vi "Update Configuration Ctls.vi"(6 "Units":refnum<vi>, 8 "error in":errorcluster, 9 "Type":refnum<vi>, 10 "selected channels":i32[](listbox)=[0], 11 "9210 in":refnum<class "9210.lvclass">) -> (0 "error out":errorcluster, 3 "9210 out":refnum<class "9210.lvclass">)   [LabVIEW 2017, in "Modules.lvlib" / "9210.lvclass"]
uses:
  9210.lvclass
  9210.lvclass/9210.ctl
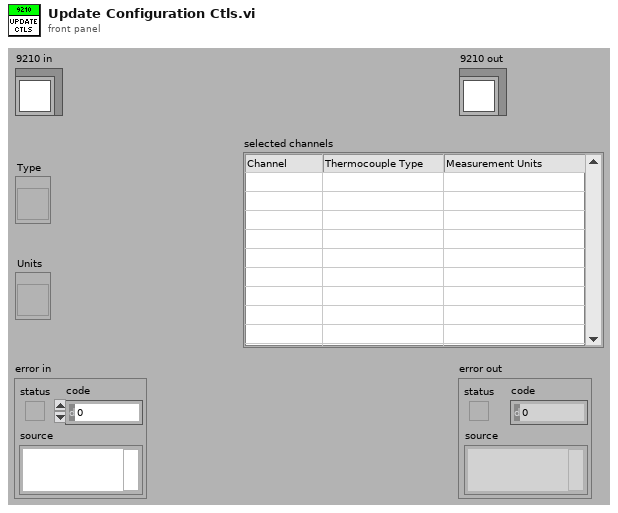
[diagram p1: front panel]
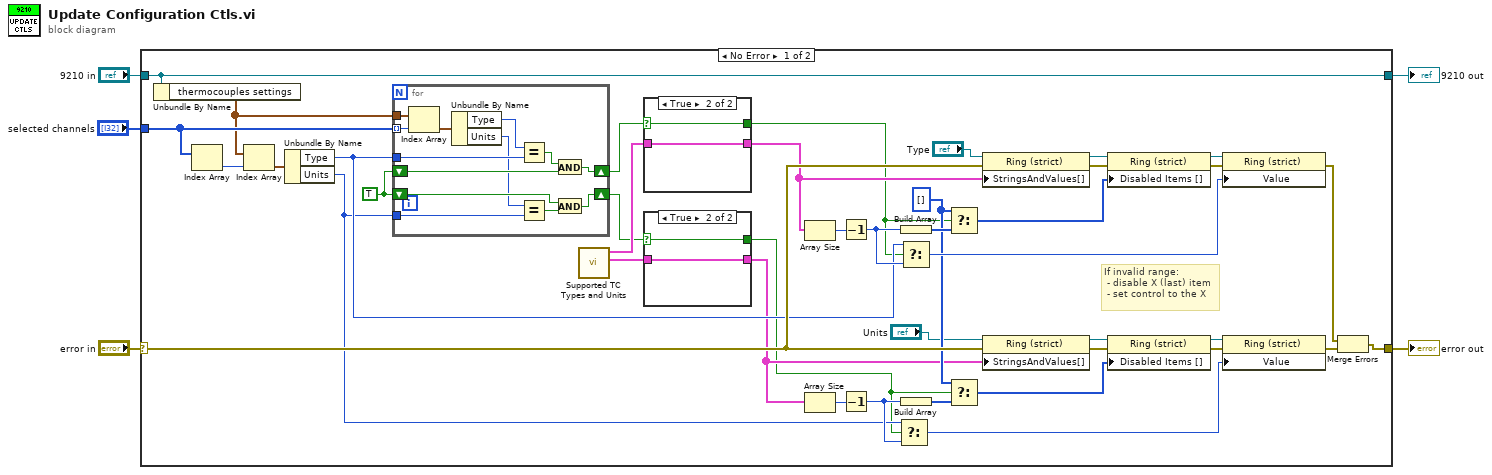
[diagram p0: block diagram]
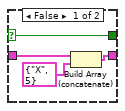
[diagram p2: hidden frame]
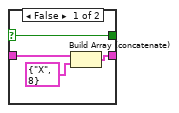
[diagram p3: hidden frame]
diagram:
  n1 = case shown="No Error" "error in" {
    selector: "error in" -> [w31 w73]
    tunnel: [w28 w73] -> w4
    tunnel: [w20 w72] -> w2
    tunnel: "9210 in" -> [w20 w72]
    tunnel: "selected channels" -> [w26 _]
    frame No Error {
      w23 = TRUE
      w19 = i32[] [] ("t")
      # "If invalid range:\n - disable X (last) item\n - set control to the X"
      n2 = Unbundle By Name(w20) -> ("thermocouples settings"=w25:cluster{"Units":u8, "Type":u8}[])
      n3 = Index Array(array=w26) -> (element=w27:i32)  [unwired: 1 in]
      n4 = Index Array(array=w25, index=w27) -> (element=w24:cluster{"Units":u8, "Type":u8})
      n5 = Unbundle By Name(w24) -> ("Type"=w22:u8, "Units"=w21:u8)
      n6 = for {
        tunnel: w26 -> [w70] mode=indexing
        tunnel: w25 -> [w71]
        tunnel: w22 -> [w69]
        shift-right: [w67] -> w18
        shift-left: w23 -> [w66]
        tunnel: w21 -> [w60]
        shift-right: [w62] -> w13
        shift-left: w23 -> [w63]
        n7 = Index Array(array=w71, index=w70) -> (element=w65:cluster{"Units":u8, "Type":u8})
        n8 = Unbundle By Name(w65) -> ("Type"=w64:u8, "Units"=w59:u8)
        n9 = Equal?(x=w64, y=w69) -> (x = y?=w68:bool)
        n10 = Equal?(x=w59, y=w60) -> (x = y?=w61:bool)
        n11 = And(x=w68, y=w66) -> (x .and. y?=w67:bool)
        n12 = And(x=w63, y=w61) -> (x .and. y?=w62:bool)
      }
      n13 = call "Supported TC Types and Units.vi"() -> ("supported temperature units"=w15:cluster{"String":string, "Value":u16}[], "supported TC types"=w17:cluster{"String":string, "Value":u16}[])  [unwired: 10 in]
      n14 = case shown="True" w18 {
        selector: w18 -> [w56 w58]
        tunnel: [w56 w58] -> w6
        tunnel: w17 -> [w55 w57]
        tunnel: [w53 w57] -> w16
        frame False {
          n15 = Build Array (concatenate)(w55, cluster{"String":string, "Value":u16} {"String"="X", "Value"=8}) -> (w53:cluster{"String":string, "Value":u16}[])
        }
        frame True {
        }
      }
      n16 = case shown="True" w13 {
        selector: w13 -> [w50 w52]
        tunnel: [w50 w52] -> w12
        tunnel: w15 -> [w49 w51]
        tunnel: [w48 w51] -> w14
        frame False {
          n17 = Build Array (concatenate)(w49, cluster{"String":string, "Value":u16} {"String"="X", "Value"=5}) -> (w48:cluster{"String":string, "Value":u16}[])
        }
        frame True {
        }
      }
      n18 = Array Size(array=w16) -> (size(s)=w37:i32)
      n19 = Array Size(array=w14) -> (size(s)=w34:i32)
      n20 = Decrement(x=w37) -> (x-1=w36:i32)
      n21 = Decrement(x=w34) -> (x-1=w35:i32)
      n22 = Select(t=w21, s=w12, f=w35) -> (s? t:f=w40:i32)
      n23 = Build Array(w36) -> (w38:i32[])
      n24 = Select(t=w22, s=w6, f=w36) -> (s? t:f=w46:i32)
      n25 = Build Array(w35) -> (w33:i32[])
      n26 = Select(t=w19, s=w6, f=w38) -> (s? t:f=w45:i32[])
      n27 = Select(t=w19, s=w12, f=w33) -> (s? t:f=w39:i32[])
      n28 = property on="Property Node" class="Ring (strict)"(reference="Type", error in=w31, "StringsAndValues[]"=w16) -> (reference out=w11:refnum<vi>, error out=w44:errorcluster)
      n29 = property on="Property Node" class="Ring (strict)"(reference="Units", error in=w31, "StringsAndValues[]"=w14) -> (reference out=w8:refnum<vi>, error out=w41:errorcluster)
      n30 = property on="Property Node" class="Ring (strict)"(reference=w11, error in=w44, "Disabled Items []"=w45) -> (reference out=w10:refnum<vi>, error out=w43:errorcluster)
      n31 = property on="Property Node" class="Ring (strict)"(reference=w8, error in=w41, "Disabled Items []"=w39) -> (reference out=w7:refnum<vi>, error out=w42:errorcluster)
      n32 = property on="Property Node" class="Ring (strict)"(reference=w10, error in=w43, "Value"=w46) -> (error out=w30:errorcluster)  [unwired: 1 out]
      n33 = property on="Property Node" class="Ring (strict)"(reference=w7, error in=w42, "Value"=w40) -> (error out=w29:errorcluster)  [unwired: 1 out]
      n34 = Merge Errors(w30, w29) -> (w28:errorcluster)
    }
    frame Error {
    }
  }
  "error out" <- w4
  "9210 out" <- w2
